vi "Decorator.vi"(10 "Component":refnum<class "Component.lvclass">, 11 "Decorator in":refnum<class "Decorator.lvclass">) -> (3 "Decorator out":refnum<class "Component.lvclass">)   [LabVIEW 2021, in "Decorator.lvclass"]
uses:
  Decorator.lvclass
  C:/PPLs/Decorator-Pattern/decorator-main/Presentation/Component/Component.lvclass
  Component/Component.lvclass
  Decorator.lvclass/Decorator.ctl
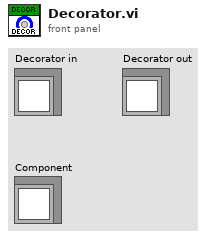
[diagram p1: front panel]
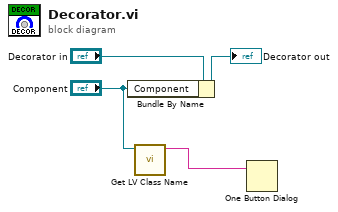
[diagram p0: block diagram]
diagram:
  n1 = Bundle By Name(cluster="Decorator in", "Component"="Component") -> (→"Decorator out":refnum<class "Decorator.lvclass">)
  n2 = call <vilib>:"Get LV Class Name.vi"("object"="Component") -> ("class name"=w2:string)  [unwired: 9 in, 1 out]
  n3 = One Button Dialog(message=w2) -> ()  [unwired: 1 in, 1 out]
